vi "Build VFH.vi"(7 "obstacle clearance (distance)":dbl, 8 "histogram in":dbl[](array[numeric]), 10 "sensor angles (radians)":dbl[](array[numeric]), 11 "sensor range (distance)":dbl[](array[numeric])) -> (0 "histogram out":dbl[](array[numeric]))   [LabVIEW 2017, in "NI_Robotics_Vector Field Histogram.lvlib"]
uses:
  <vilib>/robotics/Obstacle Avoidance/Advanced Vector Field Histogram/NI_Robotics_Vector Field Histogram.lvlib
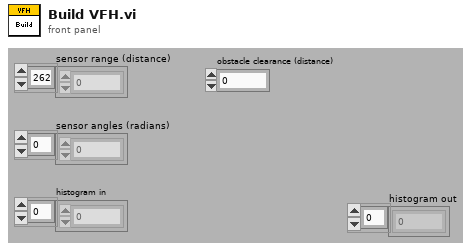
[diagram p1: front panel]
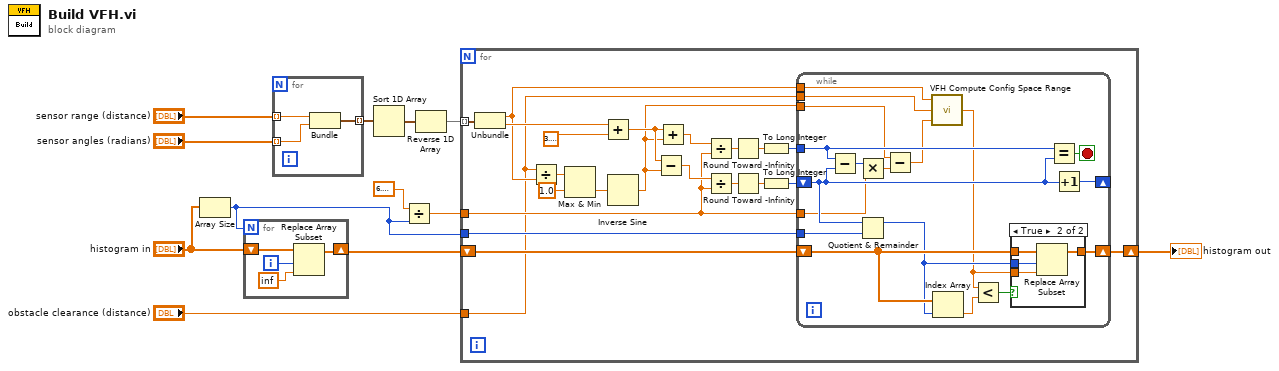
[diagram p0: block diagram]
diagram:
  n1 = Array Size(array="histogram in") -> (size(s)=w1:i32)
  n2 = for {
    N: w1 -> [_]
    shift-right: [w14] -> w3
    shift-left: "histogram in" -> [w16]
    i -> [w15]
    n3 = Replace Array Subset(array=w16, new element=inf ("new element/subarray"), index=w15) -> (w14:dbl[])
  }
  n4 = for {
    tunnel: "sensor range (distance)" -> [w17] mode=indexing
    tunnel: "sensor angles (radians)" -> [w18] mode=indexing
    tunnel: [w19] -> w7 mode=indexing
    n5 = Bundle("Numeric"=w17, "Numeric"=w18) -> (w19:cluster{"Numeric":dbl, "Numeric":dbl})  [unwired: 1 in]
  }
  n6 = Sort 1D Array(array=w7) -> (sorted array=w6:cluster{"Numeric":dbl, "Numeric":dbl}[])
  n7 = Divide(x=6.283185307179586, y=w1) -> (x/y=w9:dbl)
  n8 = Reverse 1D Array(array=w6) -> (reversed array=w4:cluster{"Numeric":dbl, "Numeric":dbl}[])
  n9 = for {
    shift-right: [w25] -> w11
    shift-left: w3 -> [w28]
    tunnel: w4 -> [w41] mode=indexing
    tunnel: "obstacle clearance (distance)" -> [w20]
    tunnel: w9 -> [w22]
    tunnel: w1 -> [w27]
    n10 = Unbundle(w41) -> ("Numeric"=w26:dbl, "Numeric"=w39:dbl)
    n11 = Divide(x=w20, y=w26) -> (x/y=w40:dbl)
    n12 = Max & Min(x=w40, y=1.0) -> (min(x,y)=w24:dbl)  [unwired: 1 out]
    n13 = Add(x=w39, y=3.141592653589793) -> (x+y=w38:dbl)
    n14 = Inverse Sine(1:w24) -> (0:w21:dbl)
    n15 = Subtract(x=w38, y=w21) -> (x-y=w36:dbl)
    n16 = Add(x=w38, y=w21) -> (x+y=w35:dbl)
    n17 = Divide(x=w35, y=w22) -> (x/y=w34:dbl)
    n18 = Divide(x=w36, y=w22) -> (x/y=w33:dbl)
    n19 = Round Toward -Infinity(1:w34) -> (0:w32:dbl)
    n20 = Round Toward -Infinity(1:w33) -> (0:w31:dbl)
    n21 = To Long Integer(number=w32) -> (32bit integer=w29:i32)
    n22 = To Long Integer(number=w31) -> (32bit integer=w30:i32)
    n23 = while {
      shift-right: [w58] -> _
      shift-left: w30 -> [w50]
      tunnel: w29 -> [w51]
      shift-right: [w57] -> w25
      shift-left: w28 -> [w54]
      tunnel: w27 -> [w53]
      tunnel: w26 -> [w45]
      tunnel: w22 -> [w48]
      tunnel: w21 -> [w46]
      tunnel: w20 -> [w44]
      stop <- w59 stop-if-true
      n24 = Subtract(x=w51, y=w50) -> (x-y=w49:i32)
      n25 = Multiply(x=w49, y=w48) -> (x*y=w47:dbl)
      n26 = Quotient & Remainder(x=w50, y=w53) -> (x-y*floor(x/y)=w52:i32)  [unwired: 1 out]
      n27 = Subtract(x=w46, y=w47) -> (x-y=w43:dbl)
      n28 = call <vilib>:"VFH Compute Config Space Range.vi"("dA (radians)"=w43, "obstacle clearance (distance)"=w44, "sensor range (distance)"=w45) -> ("config space range (distance)"=w42:dbl)
      n29 = Index Array(array=w54, index=w52) -> (element=w56:dbl)
      n30 = Less?(x=w42, y=w56) -> (x < y?=w55:bool)
      n31 = case shown="True" w55 {
        tunnel: [w60 w64] -> w57
        tunnel: w42 -> [_ w63]
        tunnel: w54 -> [w60 w62]
        tunnel: w52 -> [_ w61]
        frame False {
        }
        frame True {
          n32 = Replace Array Subset(array=w62, new element=w63, index=w61) -> (w64:dbl[])
        }
      }
      n33 = Equal?(x=w51, y=w50) -> (x = y?=w59:bool)
      n34 = Increment(x=w50) -> (x+1=w58:i32)
    }
  }
  "histogram out" <- w11
